vi "IMAQDevice.configureAcquisition.vi"(0 "i ref in":refnum<vi>, 5 "error in (no error)":errorcluster) -> (14 "i ref out":refnum<vi>, 19 "error out":errorcluster)   [LabVIEW 2014, in "IMAQDevice.lvlib"]
doc: "This VI configures the IMAQ Session. You have to execute it prior to the data aqcuisition.\n\nLicense Agreement for this software:\n\nCopyright (C)\nGesellschaft für Schwerionenforschung, GSI\nPlanckstr. 1\n64291 Darmstadt\nGermany\n\nContact: D.Beck@gsi.de \n\nThis program is free software; you can redistribute it and/or modify it under the terms of the \nGNU General Public License as published by the Free Software Foundation; either version 2 of \nthe license, or (at your option) any later version.\n\nThis program is distributed in the hope that it will be useful, but WITHOUT ANY WARRANTY; \nwithout even the implied warranty of MERCHANTABILITY or FITNESS FOR A PARTICULAR PURPOSE. See the GNU General License for more details (http://www.gnu.org).\n\nGesellschaft für Schwerionenforschung, GSI\nPlanckstr. 1, 64291 Darmstadt, Germany\nFor all questions and ideas contact: M.Richter@gsi.de, H.Brand@gsi.de or D.Beck@gsi.de.\nLast update: 16-JUN-2004"
uses:
  IMAQDevice.lvlib
  CSlibraries-extern/HGF/HGF_LVC/HGF_IMAQ/HGF_IMAQDevice/HGF_IMAQDevice.lvclass
  CSCore/CSSystem/CSSystemLib/CSSystemLib.lvlib
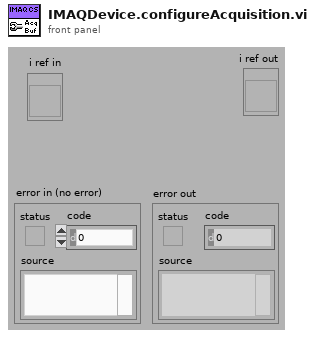
[diagram p1: front panel]
types:
  T1 = typedef "Image Type" = u32
  T2 = typedef "IMAQDevice.lvlib/IMAQDevice.i attribute.ctl" = cluster{"HGF_IMAQ.lvlib:HGF_IMAQDevice.lvclass":refnum<class "HGF_IMAQDevice.lvclass">, "Image":T3, "TimeStampID":i32, "Image IDs":i32[], "NumberOfImagesID":i32, "JPEG?":bool, "JPEGID":i32, "JPEG_ImageID":i32, "TriggerModeID":i32, "OffsetFromLeft":i32, "OffsetFromTop":i32, "HorizontalPixelPerMm":dbl, "VerticalPixelPerMm":dbl, "Grid":cluster{"1":cluster{i32, i32}, "2":cluster{i32, i32}, "3":cluster{i32, i32}, "4":cluster{i32, i32}}, "GridR":cluster{"1":cluster{dbl, dbl}, "2":cluster{dbl, dbl}, "3":cluster{dbl, dbl}, "4":cluster{dbl, dbl}}, "CameraTypeID":i32, "CameraInfos":cluster{"Camera Name-Array":string[], "own Camera Type":string}, "TakeMeasurement?":bool, "TriggerArmedID":i32, "Mirroring":i16, "Rotation":dbl}
  T3 = typedef "IMAQ Image.ctl" = refnum<image>
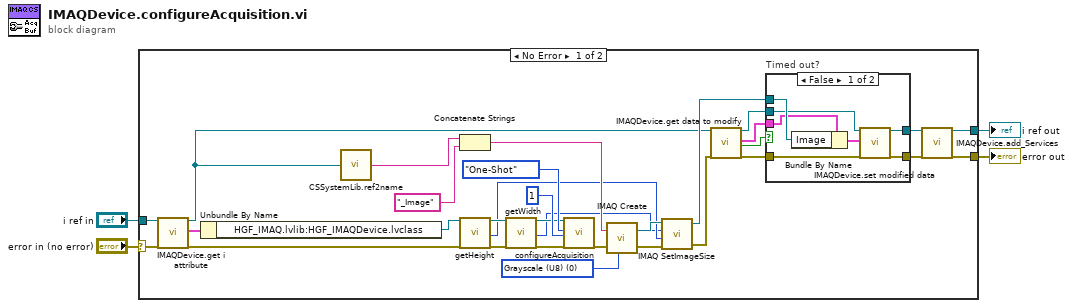
[diagram p0: block diagram]
diagram:
  n1 = case shown="No Error" "error in (no error)" {
    selector: "error in (no error)" -> [w14 w46]
    tunnel: "i ref in" -> [w13 w45]
    tunnel: [w22 w46] -> w2
    tunnel: [w24 w45] -> w1
    frame No Error {
      w33 = T1 0 items=["Grayscale (U8)", "Grayscale (I16)", "Grayscale (SGL)", "Complex (CSG)", "RGB (U32)", "HSL (U32)", "RGB (U64)", "Grayscale (U16)"] ("Image Type")
      n2 = call "IMAQDevice.get i attribute.vi"("i ref in"=w13, "error in (no error)"=w14) -> ("i ref out"=w18:refnum<vi>, "i attribute"=w21:T2, "error out"=w12:errorcluster)  [unwired: 15 in]
      n3 = Unbundle By Name(w21) -> ("HGF_IMAQ.lvlib:HGF_IMAQDevice.lvclass"=w9:refnum<class "HGF_IMAQDevice.lvclass">)
      n4 = call "CSSystemLib.ref2name.vi"("obj refnum"=w18) -> ("name"=w30:string)
      n5 = Concatenate Strings(w30, "_Image" ("string")) -> (w31:string)
      n6 = call-dynamic "getHeight.vi"("HGF_IMAQDevice in"=w9, "error in (no error)"=w12) -> ("HGF_IMAQDevice out"=w8:refnum<class "HGF_IMAQDevice.lvclass">, "Height"=w6:i32, "error out"=w11:errorcluster)  [unwired: 15 in]
      n7 = call-dynamic "getWidth.vi"("HGF_IMAQDevice in"=w8, "error in (no error)"=w11) -> ("HGF_IMAQDevice out"=w7:refnum<class "HGF_IMAQDevice.lvclass">, "Width"=w5:i32, "error out"=w10:errorcluster)  [unwired: 15 in]
      n8 = call "configureAcquisition.vi"("HGF_IMAQDevice"=w7, "Continuous?"=enum16{"One-Shot", "Continuous"}."One-Shot", "Number of buffers"=u32 1, "error in (no error)"=w10) -> ("error out"=w32:errorcluster)  [unwired: 14 in, 1 out]
      n9 = call "IMAQ Create"("Image Name"=w31, "Image Type"=w33, "error in (no error)"=w32) -> ("New Image"=w28:T3, "error out"=w26:errorcluster)  [unwired: 1 in, 1 out]
      n10 = call "IMAQ SetImageSize"("error in (no error)"=w26, "Y Resolution"=w6, "X Resolution"=w5, "Image"=w28) -> ("error out"=w20:errorcluster, "Image Out"=w27:T3)  [unwired: 1 in]
      n11 = call "IMAQDevice.get data to modify.vi"("i ref in"=w18, "error in (no error)"=w20) -> ("i ref out"=w17:refnum<vi>, "i attribute"=w16:T2, "timed out"=w15:bool, "error out"=w19:errorcluster)  [unwired: 14 in]
      n12 = case "Timed out?" shown="False" w15 {
        tunnel: w27 -> [w41 _]
        tunnel: [w40 w44] -> w25
        tunnel: [w39 w43] -> w23
        tunnel: w19 -> [w38 w43]
        tunnel: w17 -> [w37 w44]
        tunnel: w16 -> [w36 _]
        frame False {
          n13 = Bundle By Name(cluster=w36, "Image"=w41) -> (w42:T2)
          n14 = call "IMAQDevice.set modified data.vi"("i ref in"=w37, "i attribute"=w42, "error in (no error)"=w38) -> ("i ref out"=w40:refnum<vi>, "error out"=w39:errorcluster)  [unwired: 15 in]
        }
        frame True {
        }
      }
      n15 = call "IMAQDevice.add_Services.vi"("i ref in"=w25, "error in (no error)"=w23) -> ("i ref out"=w24:refnum<vi>, "error out"=w22:errorcluster)  [unwired: 16 in]
    }
    frame Error {
    }
  }
  "i ref out" <- w1
  "error out" <- w2
